vi "Front_Lifter_Function.vi"(4 "Joystick Values":T2) -> (1 "Lifter Status":T1)   [LabVIEW 2015]
uses:
  <vilib>/Rock Robotics/Network Tables/SD Read Boolean.vi
panel:
  in  "Lifter Status Def":T1
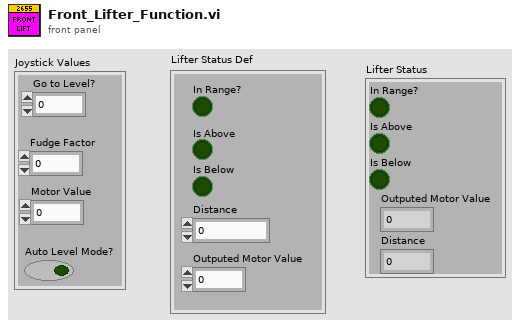
[diagram p1: front panel]
types:
  T1 = cluster{"In Range?":bool, "Is Above":bool, "Is Below":bool, "Outputed Motor Value":dbl, "Distance":dbl}
  T2 = cluster{"Go to Level?":i32, "Fudge Factor":dbl, "Auto Level Mode?":bool, "Motor Value":dbl}
  T3 = typedef "WPI_EncoderDevRef.ctl" = cluster{"DevStatus":errorcluster, "EncoderIndex":T4, "CounterIndex":T5, "DistancePerCount":dbl, "Decoding Type":T6}
  T4 = typedef "FPGA_EncoderIdx.ctl" = enum8{"Enc 0", "Enc 1", "Enc 2", "Enc 3", "Enc 4", "Enc 5", "Enc 6", "Enc 7", "Invalid"}
  T5 = typedef "FPGA_CounterCtrSystemIndex.ctl" = enum8{"Ctr 0", "Ctr 1", "Ctr 2", "Ctr 3", "Ctr 4", "Ctr 5", "Ctr 6", "Ctr 7", "Invalid"}
  T6 = typedef "WPI_EncoderType.ctl" = enum16{"1x", "2x", "4x"}
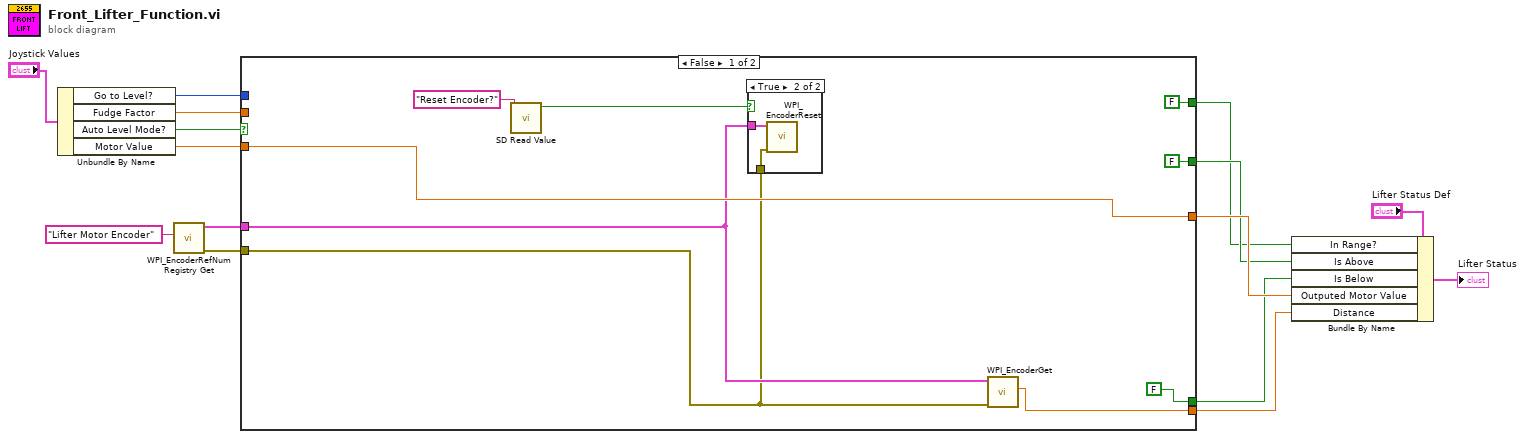
[diagram p0: block diagram]
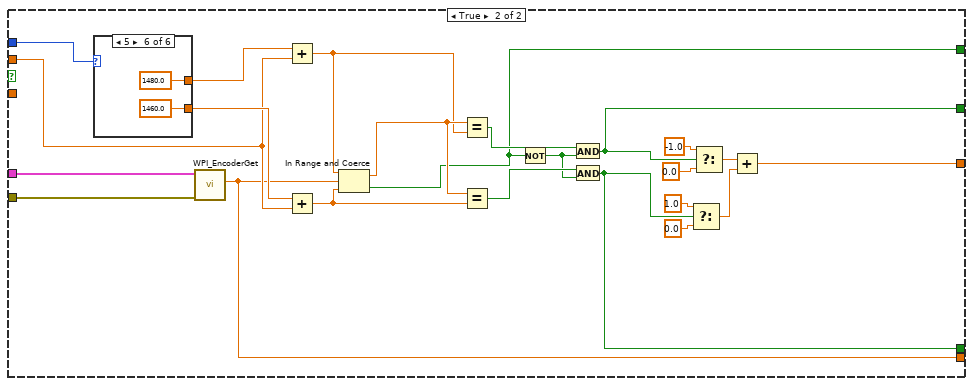
[diagram p3: hidden frame]
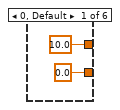
[diagram p4: hidden frame]
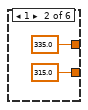
[diagram p5: hidden frame]
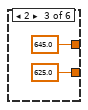
[diagram p6: hidden frame]
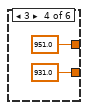
[diagram p7: hidden frame]
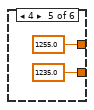
[diagram p8: hidden frame]
diagram:
  n1 = Unbundle By Name("Joystick Values") -> ("Go to Level?"=w14:i32, "Fudge Factor"=w11:dbl, "Auto Level Mode?"=w13:bool, "Motor Value"=w12:dbl)
  n2 = call <vilib>:"WPI_EncoderRefNum Registry Get.vi"("refnum name"="Lifter Motor Encoder") -> ("error out"=w1:errorcluster, "EncoderDevRef"=w2:T3)  [unwired: 9 in]
  n3 = case shown="False" w13 {
    tunnel: w12 -> [w21 _]
    tunnel: [w21 w41] -> w9
    tunnel: w14 -> [_ w40]
    tunnel: w11 -> [_ w39]
    tunnel: [w20 w38] -> w8
    tunnel: [FALSE w37] -> w7
    tunnel: [FALSE w36] -> w6
    tunnel: [FALSE w35] -> w5
    tunnel: w2 -> [w17 w34]
    tunnel: w1 -> [w16 w33]
    frame False {
      n4 = call-poly <vilib>:"SD Read Value.vi"("Name"="Reset Encoder?") -> ("Boolean"=w18:bool)  [unwired: 8 in, 2 out]
      n5 = case shown="True" w18 {
        tunnel: w17 -> [_ w26]
        tunnel: w16 -> [_ w25]
        frame False {
        }
        frame True {
          n6 = call <vilib>:"WPI_EncoderReset.vi"("error in (no error)"=w25, "EncoderDevRef"=w26) -> ()  [unwired: 8 in, 2 out]
        }
      }
      n7 = call <vilib>:"WPI_EncoderGet.vi"("error in (no error)"=w16, "EncoderDevRef"=w17) -> ("Distance"=w20:dbl)  [unwired: 4 in, 5 out]
    }
    frame True {
      n8 = case shown="5" w40 {
        tunnel: [10.0 ("upper limit") 335.0 ("upper limit") 645.0 ("upper limit") 951.0 ("upper limit") 1255.0 ("upper limit") 1480.0 ("upper limit")] -> w46
        tunnel: [0.0 ("lower Limit") 315.0 ("lower Limit") 625.0 ("lower Limit") 931.0 ("lower Limit") 1235.0 ("lower Limit") 1460.0 ("lower Limit")] -> w45
        frame 0, Default {
        }
        frame 1 {
        }
        frame 2 {
        }
        frame 3 {
        }
        frame 4 {
        }
        frame 5 {
        }
      }
      n9 = call <vilib>:"WPI_EncoderGet.vi"("error in (no error)"=w33, "EncoderDevRef"=w34) -> ("Distance"=w38:dbl)  [unwired: 4 in, 5 out]
      n10 = Add(x=w46, y=w39) -> (x+y=w43:dbl)
      n11 = Add(x=w45, y=w39) -> (x+y=w44:dbl)
      n12 = In Range and Coerce(upper limit=w43, x=w38, lower limit=w44) -> (coerced(x)=w49:dbl, In Range?=w35:bool)
      n13 = Equal?(x=w49, y=w43) -> (x = y?=w42:bool)
      n14 = Equal?(x=w49, y=w44) -> (x = y?=w48:bool)
      n15 = Not(x=w35) -> (.not. x?=w47:bool)
      n16 = And(x=w42, y=w47) -> (x .and. y?=w36:bool)
      n17 = And(x=w48, y=w47) -> (x .and. y?=w37:bool)
      n18 = Select(t=1.0, s=w37, f=0.0) -> (s? t:f=w32:dbl)
      n19 = Select(t=-1.0, s=w36, f=0.0) -> (s? t:f=w31:dbl)
      n20 = Add(x=w31, y=w32) -> (x+y=w41:dbl)
    }
  }
  n21 = Bundle By Name(cluster="Lifter Status Def", "In Range?"=w5, "Is Above"=w6, "Is Below"=w7, "Outputed Motor Value"=w9, "Distance"=w8) -> (→"Lifter Status":T1)
